vi "example 8 - child.vi"() -> ()   [LabVIEW 2020]
panel:
  in  "n-label-unvis":bool
  in  "n-label-vis":bool
  in  "m-label-vis":bool
  in  "m-label-unvis":bool
  in  "Reset":bool
  out "String":string
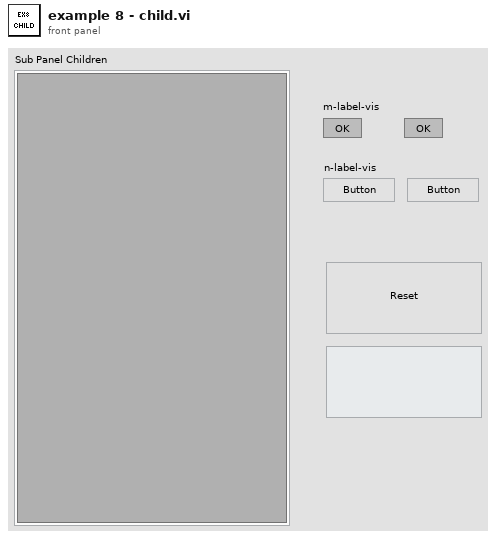
[diagram p1: front panel]
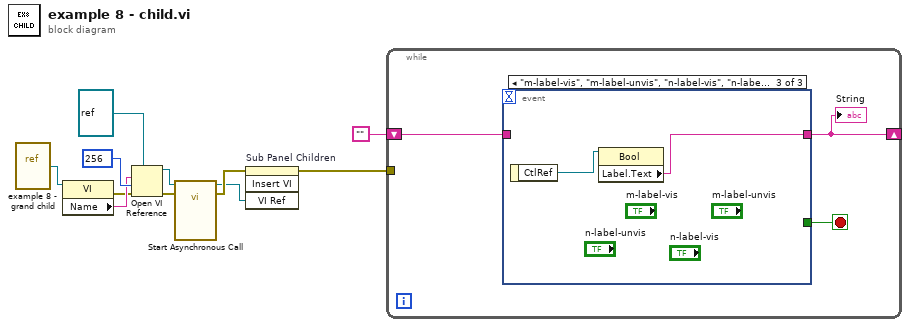
[diagram p0: block diagram]
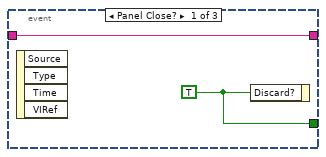
[diagram p2: hidden frame]
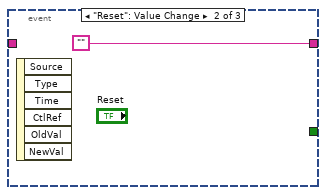
[diagram p3: hidden frame]
diagram:
  n1 = vi-ref "example 8 - grand child.vi"() -> (w7:refnum<vi>)
  n2 = property class="VI"(reference=w7) -> (error out=w5:errorcluster, "Name"=w6:string)  [unwired: 1 in, 1 out]
  n3 = Open VI Reference(type specifier VI Refnum (for type only)=refnum<vi> refnum, vi path=w6, options=256 ("call and forget"), error in (no error)=w5) -> (vi reference=w9:refnum<vi>, error out=w8:errorcluster)  [unwired: 2 in]
  n4 = call-by-ref "Start Asynchronous Call"(reference=w9, error in=w8) -> (reference out=w3:refnum<vi>, error out=w4:errorcluster)  [unwired: 12 in]
  n5 = invoke on="Sub Panel Children" class="SubPnl" method="Insert VI"(error in=w4, "VI Ref"=w3) -> (error out=w1:errorcluster)  [unwired: 2 in, 3 out]
  n6 = while {
    shift-right: [w12] -> _
    shift-left: "" -> [w13]
    tunnel: w1 -> [_]
    stop <- w14 stop-if-true
    n7 = event shown="[2] \"m-label-vis\", \"m-label-unvis\", \"n-label-vis\", \"n-label-unvis\": Value Change" {
      selector: _ -> [_ _ _]
      dyn-events: _ -> [_ _ _]
      timeout: _ -> [_ _ _]
      tunnel: [w16 _ _] -> w14
      tunnel: [w15 "" w18] -> w12
      tunnel: w13 -> [w15 _ _]
      event Panel Close? {
        w16 = TRUE
        n8 = event-data() -> ()  [unwired: 1 in, 4 out]
        n9 = event-data("Discard?"=w16) -> ()  [unwired: 1 in, 1 out]
      }
      event "Reset": Value Change {
        n10 = event-data() -> ()  [unwired: 1 in, 6 out]
      }
      event "m-label-vis", "m-label-unvis", "n-label-vis", "n-label-unvis": Value Change {
        n11 = event-data() -> ("CtlRef"=w19:refnum<vi>)  [unwired: 1 in]
        n12 = property class="Bool"(reference=w19) -> ("Label.Text"=w18:string)  [unwired: 1 in, 2 out]
      }
    }
    "String" <- w12
  }
